vi "ClusterSimpleExample.vi"() -> ()   [LabVIEW 2019]
panel:
  out "Ebike":T1
  out "Ranger":T1
  in  "Cycle":T1
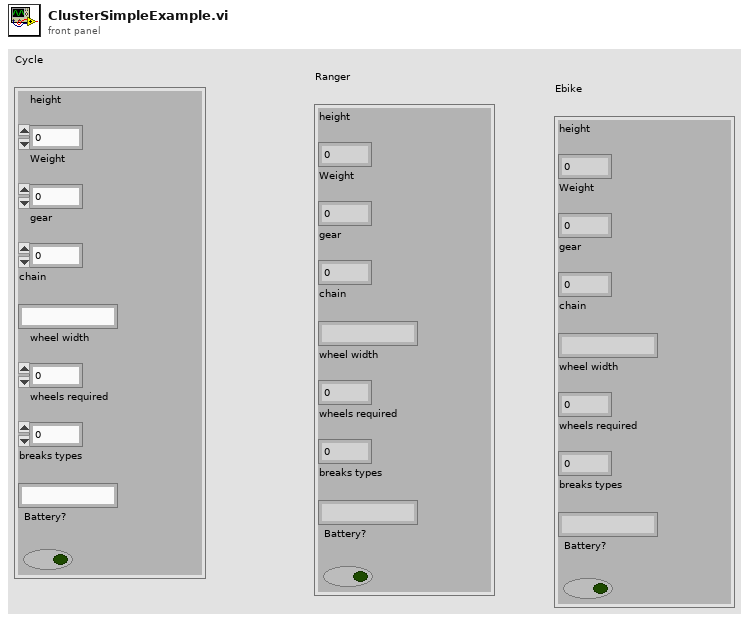
[diagram p1: front panel]
types:
  T1 = cluster{"height":u8, "Weight":u8, "gear":u8, "chain":string, "wheel width":u8, "wheels required":u8, "breaks types":string, "Battery?":bool}
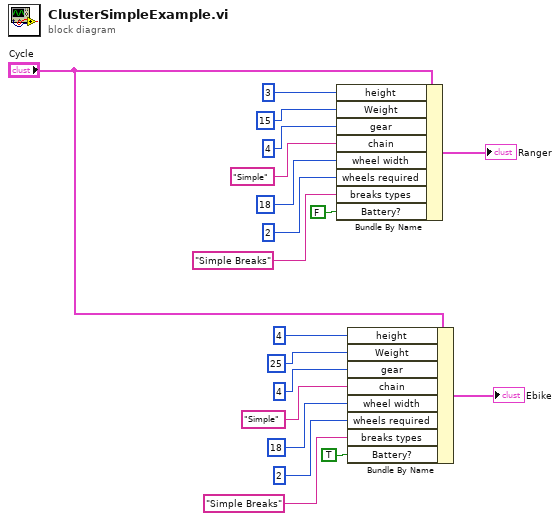
[diagram p0: block diagram]
diagram:
  n1 = Bundle By Name(cluster="Cycle", "height"=u8 3, "Weight"=u8 15, "gear"=u8 4, "chain"="Simple", "wheel width"=u8 18, "wheels required"=u8 2, "breaks types"="Simple Breaks", "Battery?"=FALSE) -> (→"Ranger":T1)
  n2 = Bundle By Name(cluster="Cycle", "height"=u8 4, "Weight"=u8 25, "gear"=u8 4, "chain"="Simple", "wheel width"=u8 18, "wheels required"=u8 2, "breaks types"="Simple Breaks", "Battery?"=TRUE) -> (→"Ebike":T1)
